vi "Str2Num.vi"(1 "InputString":string="25" caption="Input String") -> (0 "Array":dbl[](array[numeric]))   [LabVIEW 2011]
uses:
  <vilib>/regexp/Match Regular Expression.xnode
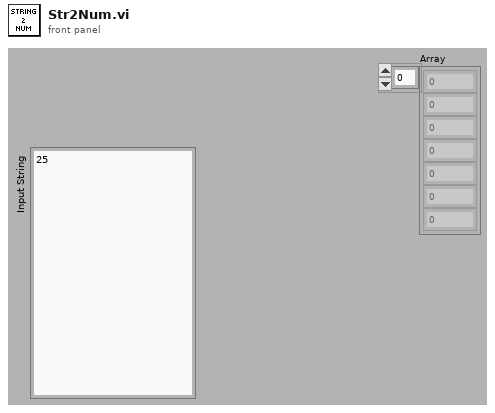
[diagram p1: front panel]
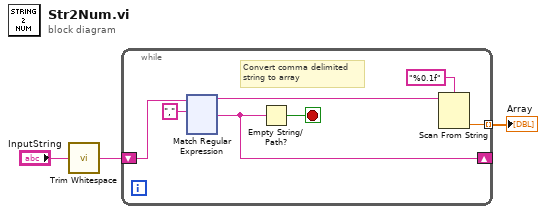
[diagram p0: block diagram]
diagram:
  n1 = call <vilib>:"Trim Whitespace.vi"("string"="InputString") -> ("trimmed string"=w2:string)  [unwired: 1 in]
  n2 = while {
    shift-right: [w5] -> _
    shift-left: w2 -> [w9]
    tunnel: [w7] -> w1 mode=indexing
    stop <- w4 stop-if-true
    # "Convert comma delimited\nstring to array"
    n3 = xnode "Match Regular Expression"("input string"=w9, "regular expression"=",") -> ("before match"=w8:string, "after match"=w5:string)  [unwired: 4 in, 3 out]
    n4 = Empty String/Path?(string/path=w5) -> (empty?=w4:bool)
    n5 = Scan From String(format string="%0.1f", input string=w8) -> (output 1=w7:dbl)  [unwired: 3 in, 3 out]
  }
  "Array" <- w1
